vi "Update POV State.vi"(8 "error in (no error)":errorcluster, 10 "POVs":i16[](array[numeric]), 11 "Joystick in":refnum<class "Joystick.lvclass">) -> (0 "error out":errorcluster, 3 "Joystick out":refnum<class "Joystick.lvclass">)   [LabVIEW 2014, in "Joystick.lvlib" / "Joystick.lvclass"]
uses:
  Joystick.lvclass
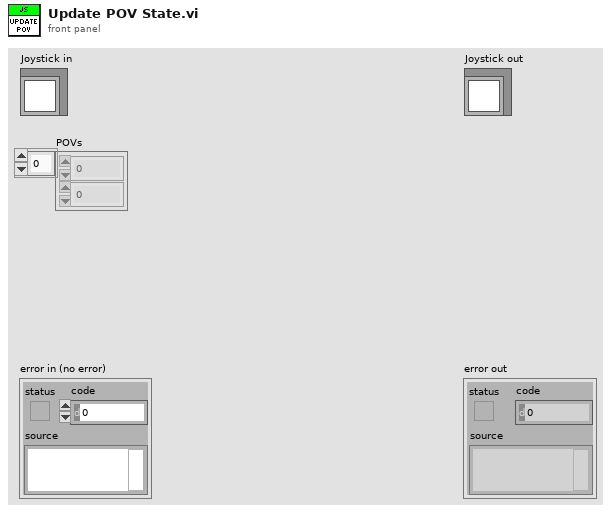
[diagram p1: front panel]
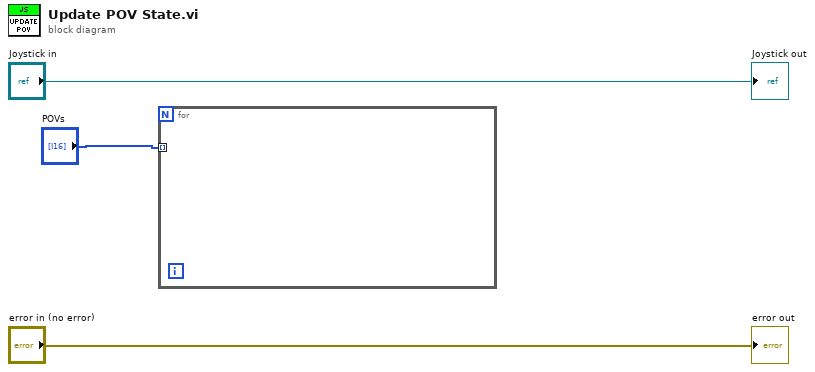
[diagram p0: block diagram]
diagram:
  n1 = for {
    tunnel: "POVs" -> [_] mode=indexing
  }
  "error out" <- "error in (no error)"
  "Joystick out" <- "Joystick in"
